vi "Read Control Width.vi"(8 "error in":errorcluster, 11 "Control in":refnum<vi>) -> (0 "error out":errorcluster, 2 "Width":u32, 3 "Control":refnum<vi>)   [LabVIEW 2020, in "VolatusGUIEditorCore.lvlib"]
uses:
  VolatusGUIEditorCore.lvlib
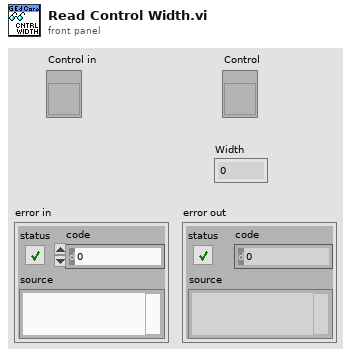
[diagram p1: front panel]
types:
  T1 = typedef "LVBoundsTypeDef.ctl" = cluster{"Width":u32, "Height":u32}
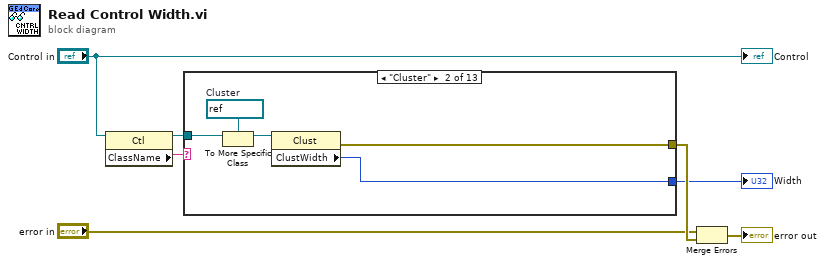
[diagram p0: block diagram]
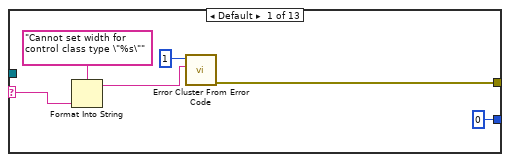
[diagram p2: hidden frame]
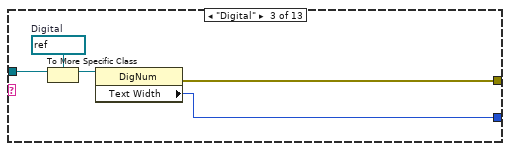
[diagram p3: hidden frame]
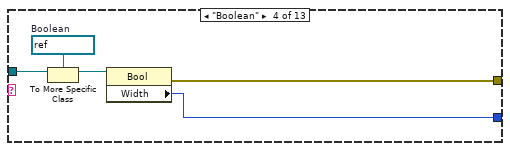
[diagram p4: hidden frame]
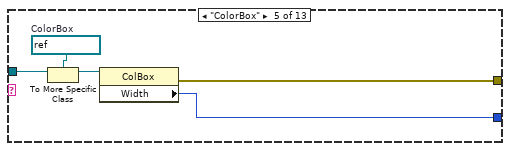
[diagram p5: hidden frame]
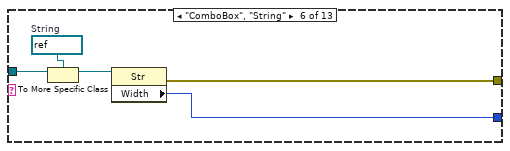
[diagram p6: hidden frame]
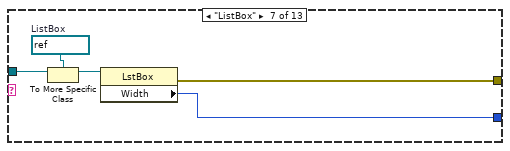
[diagram p7: hidden frame]
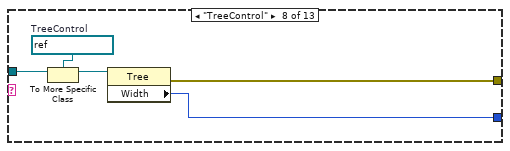
[diagram p8: hidden frame]
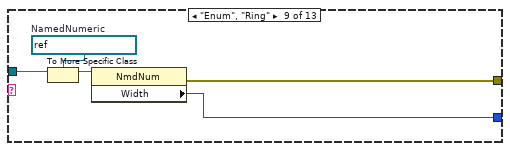
[diagram p9: hidden frame]
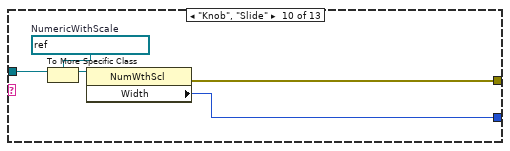
[diagram p10: hidden frame]
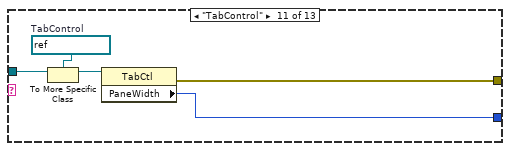
[diagram p11: hidden frame]
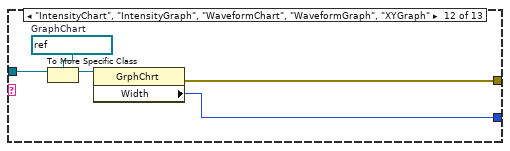
[diagram p12: hidden frame]
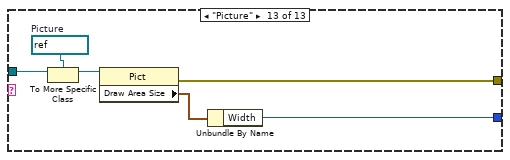
[diagram p13: hidden frame]
diagram:
  n1 = property class="Ctl"(reference="Control in") -> (reference out=w6:refnum<vi>, "ClassName"=w7:string)  [unwired: 1 in, 1 out]
  n2 = case shown="\"Cluster\"" w7 {
    selector: w7 -> [w10 _ _ _ _ _ _ _ _ _ _ _ _]
    tunnel: w6 -> [_ w18 w23 w28 w33 w38 w43 w48 w53 w58 w63 w68 w74]
    tunnel: [w13 w15 w20 w25 w30 w35 w40 w45 w50 w55 w60 w65 w71] -> w4
    tunnel: [u32 0 ("Width") w14 w19 w24 w29 w34 w39 w44 w49 w54 w59 w64 w69] -> w1
    frame Default {
      n3 = Format Into String(format string="Cannot set width for control class type \"%s\"", w10) -> (resulting string=w9:string)  [unwired: 2 in, 1 out]
      n4 = call <vilib>:"Error Cluster From Error Code.vi"("error message (\"\")"=w9, "error code (0)"=1) -> ("error out"=w13:errorcluster)  [unwired: 7 in]
    }
    frame "Cluster" {
      w17 = refnum<vi> refnum  # Cluster
      n5 = To More Specific Class(target class=w17, reference=w18) -> (specific class reference=w16:refnum<vi>)  [unwired: 1 in, 1 out]
      n6 = property class="Clust"(reference=w16) -> (error out=w15:errorcluster, "ClustWidth"=w14:u32)  [unwired: 1 in, 1 out]
    }
    frame "Digital" {
      w22 = refnum<vi> refnum  # Digital
      n7 = To More Specific Class(target class=w22, reference=w23) -> (specific class reference=w21:refnum<vi>)  [unwired: 1 in, 1 out]
      n8 = property class="DigNum"(reference=w21) -> (error out=w20:errorcluster, "Text Width"=w19:u32)  [unwired: 1 in, 1 out]
    }
    frame "Boolean" {
      w27 = refnum<vi> refnum  # Boolean
      n9 = To More Specific Class(target class=w27, reference=w28) -> (specific class reference=w26:refnum<vi>)  [unwired: 1 in, 1 out]
      n10 = property class="Bool"(reference=w26) -> (error out=w25:errorcluster, "Width"=w24:u32)  [unwired: 1 in, 1 out]
    }
    frame "ColorBox" {
      w32 = refnum<vi> refnum  # ColorBox
      n11 = To More Specific Class(target class=w32, reference=w33) -> (specific class reference=w31:refnum<vi>)  [unwired: 1 in, 1 out]
      n12 = property class="ColBox"(reference=w31) -> (error out=w30:errorcluster, "Width"=w29:u32)  [unwired: 1 in, 1 out]
    }
    frame "ComboBox", "String" {
      w37 = refnum<vi> refnum  # String
      n13 = To More Specific Class(target class=w37, reference=w38) -> (specific class reference=w36:refnum<vi>)  [unwired: 1 in, 1 out]
      n14 = property class="Str"(reference=w36) -> (error out=w35:errorcluster, "Width"=w34:u32)  [unwired: 1 in, 1 out]
    }
    frame "ListBox" {
      w42 = refnum<vi> refnum  # ListBox
      n15 = To More Specific Class(target class=w42, reference=w43) -> (specific class reference=w41:refnum<vi>)  [unwired: 1 in, 1 out]
      n16 = property class="LstBox"(reference=w41) -> (error out=w40:errorcluster, "Width"=w39:u32)  [unwired: 1 in, 1 out]
    }
    frame "TreeControl" {
      w47 = refnum<vi> refnum  # TreeControl
      n17 = To More Specific Class(target class=w47, reference=w48) -> (specific class reference=w46:refnum<vi>)  [unwired: 1 in, 1 out]
      n18 = property class="Tree"(reference=w46) -> (error out=w45:errorcluster, "Width"=w44:u32)  [unwired: 1 in, 1 out]
    }
    frame "Enum", "Ring" {
      w52 = refnum<vi> refnum  # NamedNumeric
      n19 = To More Specific Class(target class=w52, reference=w53) -> (specific class reference=w51:refnum<vi>)  [unwired: 1 in, 1 out]
      n20 = property class="NmdNum"(reference=w51) -> (error out=w50:errorcluster, "Width"=w49:u32)  [unwired: 1 in, 1 out]
    }
    frame "Knob", "Slide" {
      w57 = refnum<vi> refnum  # NumericWithScale
      n21 = To More Specific Class(target class=w57, reference=w58) -> (specific class reference=w56:refnum<vi>)  [unwired: 1 in, 1 out]
      n22 = property class="NumWthScl"(reference=w56) -> (error out=w55:errorcluster, "Width"=w54:u32)  [unwired: 1 in, 1 out]
    }
    frame "TabControl" {
      w62 = refnum<vi> refnum  # TabControl
      n23 = To More Specific Class(target class=w62, reference=w63) -> (specific class reference=w61:refnum<vi>)  [unwired: 1 in, 1 out]
      n24 = property class="TabCtl"(reference=w61) -> (error out=w60:errorcluster, "PaneWidth"=w59:u32)  [unwired: 1 in, 1 out]
    }
    frame "IntensityChart", "IntensityGraph", "WaveformChart", "WaveformGraph", "XYGraph" {
      w67 = refnum<vi> refnum  # GraphChart
      n25 = To More Specific Class(target class=w67, reference=w68) -> (specific class reference=w66:refnum<vi>)  [unwired: 1 in, 1 out]
      n26 = property class="GrphChrt"(reference=w66) -> (error out=w65:errorcluster, "Width"=w64:u32)  [unwired: 1 in, 1 out]
    }
    frame "Picture" {
      w73 = refnum<vi> refnum  # Picture
      n27 = To More Specific Class(target class=w73, reference=w74) -> (specific class reference=w72:refnum<vi>)  [unwired: 1 in, 1 out]
      n28 = property class="Pict"(reference=w72) -> (error out=w71:errorcluster, "Draw Area Size"=w70:T1)  [unwired: 1 in, 1 out]
      n29 = Unbundle By Name(w70) -> ("Width"=w69:u32)
    }
  }
  "Width" <- w1
  n30 = Merge Errors("error in", w4) -> (→"error out":errorcluster)
  "Control" <- "Control in"
